vi "main_2.vi"() -> ()   [LabVIEW 2024]
uses:
  <vilib>/addons/_JKI.lib/REST Client/classes/REST Client/REST Client.lvclass
  D:/github/CarProject/UI/typeDef/dataCluster.ctl
panel:
  out "angle":dbl
  out "Przeszkoda":dbl
  out "mapa":picture
  out "Char":i16
  out "Kierunek":dbl(knob) scale=0.0..360.0
  out "Response body":string
  in  "stop":bool
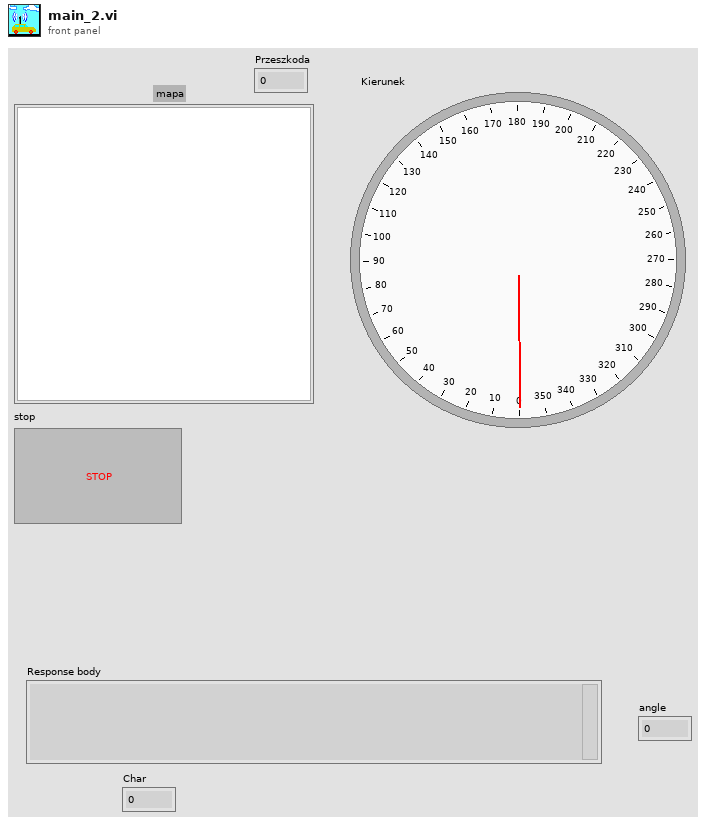
[diagram p1: front panel]
types:
  T1 = typedef "dataCluster.ctl" = cluster{"angle":dbl, "turn_left?":bool, "turn_right?":bool, "forward?":bool, "backward?":bool, "stop?":bool, "distance":dbl}
  T2 = cluster{"Width":u16, "Style":enum32{"Solid", "Dash", "Dot", "DashDot", "DashDotDot"}}
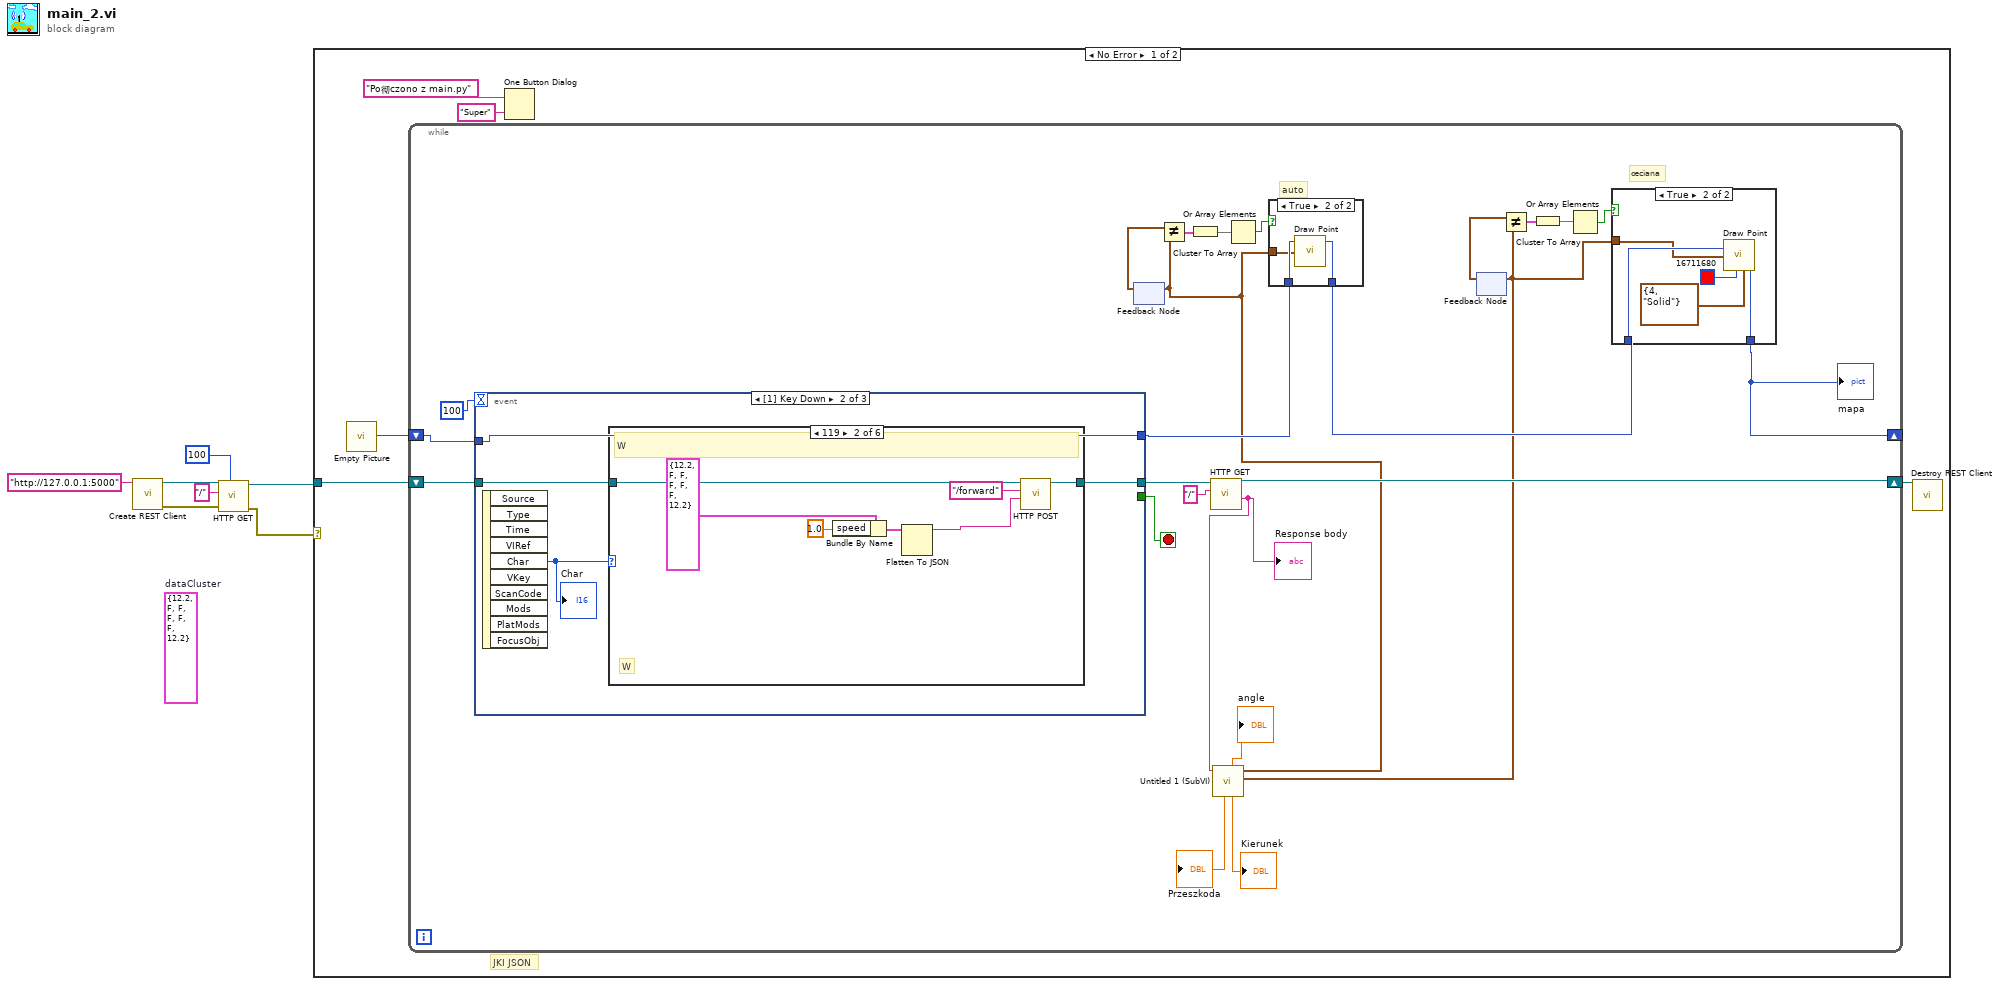
[diagram p0: block diagram]
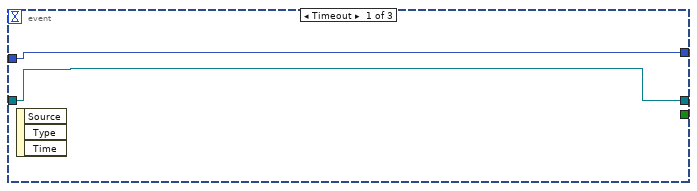
[diagram p4: hidden frame]
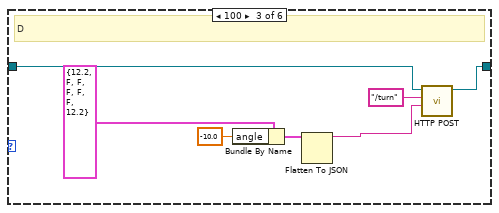
[diagram p6: hidden frame]
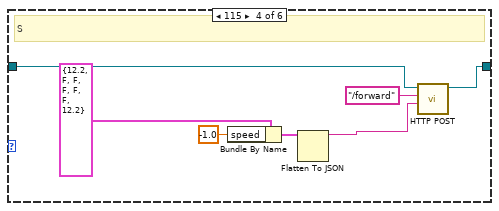
[diagram p7: hidden frame]
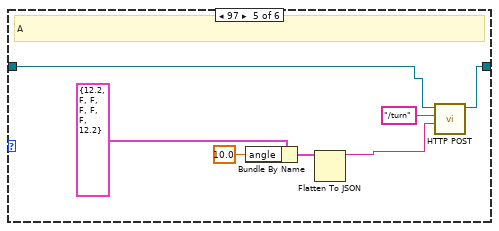
[diagram p8: hidden frame]
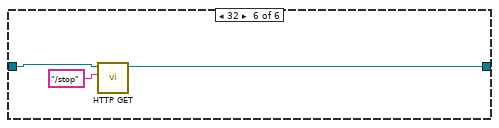
[diagram p9: hidden frame]
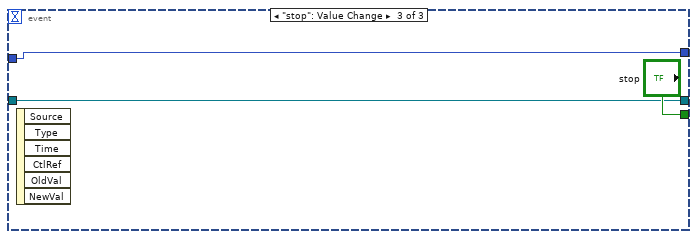
[diagram p10: hidden frame]
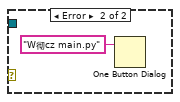
[diagram p11: hidden frame]
diagram:
  (unwired) T1 {"angle"=12.2, "turn_left?"=FALSE, "turn_right?"=FALSE, "forward?"=FALSE, "backward?"=FALSE, "stop?"=FALSE, "distance"=12.2}  # dataCluster
  n1 = call <vilib>:"Create REST Client.vi"("Base URL"="http://127.0.0.1:5000") -> ("error out"=w3:errorcluster, "REST Client out"=w6:refnum<class "REST Client.lvclass">)  [unwired: 9 in]
  n2 = call-dynamic "HTTP GET.vi"("timeout (0 = Use Default)"=100, "error in (no error)"=w3, "Path"="/", "REST Client in"=w6) -> ("error out"=w5:errorcluster, "REST Client out"=w4:refnum<class "REST Client.lvclass">)  [unwired: 2 in, 4 out]
  n3 = case shown="No Error" w5 {
    tunnel: w4 -> [w12 _]
    frame No Error {
      # "JKI JSON"
      n4 = call "Empty Picture"() -> ("empty picture"=w8:picture)
      n5 = while {
        shift-right: [w30] -> w11
        shift-left: w12 -> [w34]
        shift-right: [w17] -> _
        shift-left: w8 -> [w29]
        stop <- w36 stop-if-true
        # "œciana"
        # "auto"
        n6 = event shown="[1] Key Down" {
          selector: _ -> [_ _ _]
          dyn-events: _ -> [_ _ _]
          timeout: 100 -> [_ _ _]
          tunnel: [_ _ "stop"] -> w36
          tunnel: [w48 w50 w86] -> w31
          tunnel: w34 -> [w48 w51 w86]
          tunnel: w29 -> [w47 w49 w85]
          tunnel: [w47 w49 w85] -> w23
          event Timeout {
            n7 = event-data() -> ()  [unwired: 1 in, 3 out]
          }
          event Key Down {
            n8 = event-data() -> ("Char"=w52:i16)  [unwired: 1 in, 9 out]
            "Char" <- w52
            n9 = case shown="119" w52 {
              tunnel: w51 -> [w53 w60 w61 w69 w75 w83]
              tunnel: [w53 w59 w62 w68 w76 w82] -> w50
              frame 0, Default {
              }
              frame 119 {
                # "W"
                # "W"
                n10 = Bundle By Name(cluster=T1 {"angle"=12.2, "turn_left?"=FALSE, "turn_right?"=FALSE, "forward?"=FALSE, "backward?"=FALSE, "stop?"=FALSE, "distance"=12.2} ("dataCluster"), "speed"=1.0) -> (w56:T1)
                n11 = Flatten To JSON(anything=w56) -> (JSON string=w57:string)  [unwired: 2 in, 1 out]
                n12 = call-dynamic "HTTP POST.vi"("Request body"=w57, "Path"="/forward", "REST Client in"=w60) -> ("REST Client out"=w59:refnum<class "REST Client.lvclass">)  [unwired: 3 in, 5 out]
              }
              frame 100 {
                # "D"
                n13 = Bundle By Name(cluster=T1 {"angle"=12.2, "turn_left?"=FALSE, "turn_right?"=FALSE, "forward?"=FALSE, "backward?"=FALSE, "stop?"=FALSE, "distance"=12.2} ("dataCluster"), "angle"=-10.0 ("speed")) -> (w67:T1)
                n14 = Flatten To JSON(anything=w67) -> (JSON string=w66:string)  [unwired: 2 in, 1 out]
                n15 = call-dynamic "HTTP POST.vi"("Request body"=w66, "Path"="/turn", "REST Client in"=w61) -> ("REST Client out"=w62:refnum<class "REST Client.lvclass">)  [unwired: 3 in, 5 out]
              }
              frame 115 {
                # "S"
                n16 = Bundle By Name(cluster=T1 {"angle"=12.2, "turn_left?"=FALSE, "turn_right?"=FALSE, "forward?"=FALSE, "backward?"=FALSE, "stop?"=FALSE, "distance"=12.2} ("dataCluster"), "speed"=-1.0) -> (w73:T1)
                n17 = Flatten To JSON(anything=w73) -> (JSON string=w74:string)  [unwired: 2 in, 1 out]
                n18 = call-dynamic "HTTP POST.vi"("Request body"=w74, "Path"="/forward", "REST Client in"=w69) -> ("REST Client out"=w68:refnum<class "REST Client.lvclass">)  [unwired: 3 in, 5 out]
              }
              frame 97 {
                # "A"
                n19 = Bundle By Name(cluster=T1 {"angle"=12.2, "turn_left?"=FALSE, "turn_right?"=FALSE, "forward?"=FALSE, "backward?"=FALSE, "stop?"=FALSE, "distance"=12.2} ("dataCluster"), "angle"=10.0 ("speed")) -> (w80:T1)
                n20 = Flatten To JSON(anything=w80) -> (JSON string=w81:string)  [unwired: 2 in, 1 out]
                n21 = call-dynamic "HTTP POST.vi"("Request body"=w81, "Path"="/turn", "REST Client in"=w75) -> ("REST Client out"=w76:refnum<class "REST Client.lvclass">)  [unwired: 3 in, 5 out]
              }
              frame 32 {
                n22 = call-dynamic "HTTP GET.vi"("Path"="/stop", "REST Client in"=w83) -> ("REST Client out"=w82:refnum<class "REST Client.lvclass">)  [unwired: 4 in, 5 out]
              }
            }
          }
          event "stop": Value Change {
            n23 = event-data() -> ()  [unwired: 1 in, 6 out]
          }
        }
        n24 = feedback #1() -> (w25:cluster{dbl, dbl})  [unwired: 1 in]
        n25 = call-dynamic "HTTP GET.vi"("Path"="/", "REST Client in"=w31) -> ("Response body"=w33:string, "REST Client out"=w30:refnum<class "REST Client.lvclass">)  [unwired: 4 in, 4 out]
        "Response body" <- w33
        n26 = call "Untitled 1 (SubVI).vi"("Response body"=w33) -> ("Cluster"=w18:cluster{dbl, dbl}, "Cluster 2"=w22:cluster{dbl, dbl}, "Gauge"=→"Kierunek":dbl, "angle"=→"angle":dbl, "Przeszkoda"=→"Przeszkoda":dbl)  [unwired: 5 in, 1 out]
        n27 = feedback-in #1(w22) -> ()
        n28 = Not Equal?(x=w25, y=w22) -> (x != y?=w24:cluster{bool, bool})
        n29 = Cluster To Array(cluster=w24) -> (array=w16:bool[])
        n30 = Or Array Elements(Boolean array=w16) -> (logical OR=w15:bool)
        n31 = case shown="True" w15 {
          tunnel: w23 -> [w43 w46]
          tunnel: w22 -> [_ w45]
          tunnel: [w43 w44] -> w19
          frame False {
          }
          frame True {
            n32 = call <vilib>:"Draw Point.vi"("picture"=w46, "point(x,y)"=w45) -> ("new picture"=w44:picture)  [unwired: 7 in]
          }
        }
        n33 = feedback #2() -> (w20:cluster{dbl, dbl})  [unwired: 1 in]
        n34 = feedback-in #2(w18) -> ()
        n35 = Not Equal?(x=w20, y=w18) -> (x != y?=w21:cluster{bool, bool})
        n36 = Cluster To Array(cluster=w21) -> (array=w14:bool[])
        n37 = Or Array Elements(Boolean array=w14) -> (logical OR=w13:bool)
        n38 = case shown="True" w13 {
          tunnel: w18 -> [_ w38]
          tunnel: w19 -> [w37 w42]
          tunnel: [w37 w39] -> w17
          frame False {
          }
          frame True {
            n39 = call <vilib>:"Draw Point.vi"("picture"=w42, "point(x,y)"=w38, "color(black)"=u32 16711680, "pen"=T2 {"Width"=4, "Style"=enum."Solid"}) -> ("new picture"=w39:picture)  [unwired: 5 in]
          }
        }
        "mapa" <- w17
      }
      n40 = One Button Dialog(message="Po彻czono z main.py", button name ("OK")="Super") -> ()  [unwired: 1 out]
      n41 = call-dynamic "Destroy REST Client.vi"("REST Client in"=w11) -> ()  [unwired: 10 in, 1 out]
    }
    frame Error {
      n42 = One Button Dialog(message="W彻cz main.py") -> ()  [unwired: 1 in, 1 out]
    }
  }
